vi "WritetoFile.vi"(1 "text":string, 2 "Path":path) -> (0 "error out":errorcluster)   [LabVIEW 2013]
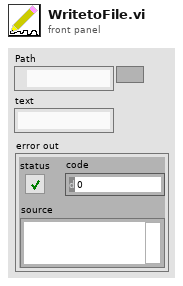
[diagram p1: front panel]
types:
  T1 = enum16{"open", "replace", "create", "open or create", "replace or create", "replace or create with confirmation"}
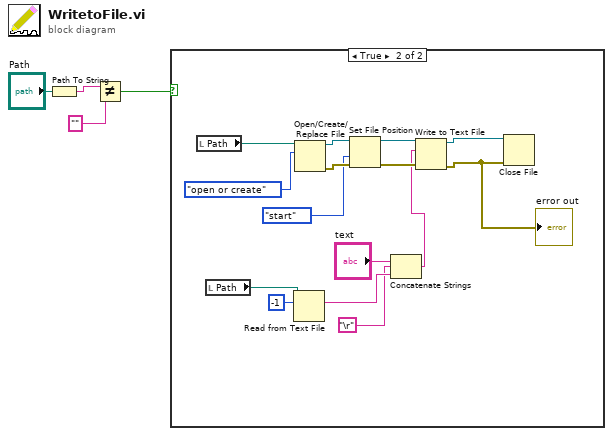
[diagram p0: block diagram]
diagram:
  n1 = Path To String(path="Path") -> (string=w3:string)
  n2 = Not Equal?(x=w3, y="") -> (x != y?=w1:bool)
  n3 = case shown="True" w1 {
    frame False {
    }
    frame True {
      n4 = local read "Path"() -> (w7:path)
      n5 = local read "Path"() -> (w11:path)
      n6 = Read from Text File(file (use dialog)=w11, count=-1) -> (text=w6:string)  [unwired: 2 in, 3 out]
      n7 = Open/Create/Replace File(file path (use dialog)=w7, operation (0:open)=T1."open or create") -> (refnum out=w18:refnum<file>, error out=w17:errorcluster)  [unwired: 4 in, 1 out]
      n8 = Set File Position(refnum=w18, from (0:start)=enum16{"start", "end", "current"}."start", error in=w17) -> (refnum out=w15:refnum<file>, error out=w14:errorcluster)  [unwired: 1 in]
      n9 = Concatenate Strings("text", "\r", w6) -> (w8:string)
      n10 = Write to Text File(file (use dialog)=w15, text=w8, error in=w14) -> (refnum out=w13:refnum<file>, error out=w12:errorcluster)  [unwired: 1 in, 1 out]
      "error out" <- w12
      n11 = Close File(refnum=w13, error in=w12) -> ()  [unwired: 2 out]
    }
  }
